vi "CA Spectra.vi"(2 "Header In":T1={"header info"={"Header"="", "Head length"=0}, "A/D info"={"# rf points per line"=0, "# lines per scan"=0, "sample rate MHz"=0, "# A/D bits"=0, "# bytes per A/D"=0, "TGC Flag"=0, "A/D Type"=""}, "Tranducer Info"={"bandwidth"=0.0, "center freq"=0.0, "start freq"=0.0, "ID"=0}, "Scan Info"={"delay"=0.0, "pivot distance"=0.0, "sector scan angle"=0.0, "operator"="", "Scan Mode"="", "location"=""}, "Time/Date Info"={"date"="", "time"=""}, "RF Info"={"RF file name"="", "RF file att"="", "RF cal file name"="", "RF cal file att"=""}, "Patient Info"={"ID"="", "extended ID"="", "age"=0, "sex"="", "previously\nscanned"="", "PSA"=0.0, "LOS"=1, "Ethnicty 2"=3, "Race"=3}, "Tissue Type"={"organ"=0, "disease type"=0, "disease location"=0, "IQ_pts"=0, "RcvBuffer"=0, "RcvFrame"=0, "IQBuff"=0, "IQFrame"=0, "IQPage"=0}, "Votage scaling"={"Digitizer (dB)"=0.0, "Gain (dB)"=0.0, "Atten (dB)"=0.0}, "Comment"="", "Misc Info"={"avg num"=0, "c speed"=0, "Div By or SF zones"=0, "XMIT CHS"=0, "RCV CHS"=0, "Xmit angle"=0.0}, "Therapy Parameters"={"Theraputic Freq (MHz)"=0.1, "Time on (s)"=1.0, "Therapy amplitude (mV)"=50.0, "Lines Before"=20, "Lines After"=80}, "Scan Settings"={"Energy (uJ or V)"=0, "Damp (Ohm) or Fc"=0, "HP Filt (KHz)"=0, "LP Filt (MHz)"=0, "Gain (db)"=0, "prf (kHz)"=0.0, "Distance between\nscan lines (um)"=0, "Distance between\nscan planes (um)"=0, "Scan line gap (um)"=0.0, "Scan plane gap (um)"=0.0}, "Compression Parameters"={"F1 (MHz)"=0.0, "F2 (MHz)"=0.0, "% taper"=0.0, "duration"=0.0}, "Patient Info Xtra"={"First Name"="", "Last Name"="", "Notes"=""}, "ROI Box"=[]} {"Compression Parameters"."% taper" min=50 max=1000 format="%.2f"; "Compression Parameters"."F2 (MHz)" format="%.3f"; "Compression Parameters"."F1 (MHz)" format="%.3f"; "Scan Settings"."prf (kHz)" format="%.2f"; "Therapy Parameters"."Therapy amplitude (mV)" min=50 max=1000 format="%.2f"; "Therapy Parameters"."Time on (s)" format="%.3f"; "Therapy Parameters"."Theraputic Freq (MHz)" format="%.3f"; "Patient Info"."Race" items=["Am Ind or Alaska", "Asian", "Hawaiian, Pac Isl", "Black or Afr Amer", "White", "more than one race", "unknown"]; "Patient Info"."Ethnicty 2" items=["Hispanic", "Non-Hispanic", "unknown"]; "Patient Info"."LOS" items=["1", "2", "3", "4", "5"]; "Patient Info"."PSA" format="%.1f"; "Scan Info"."delay" format="%.2f"; "Scan Info"."pivot distance" format="%.2f"; "Scan Info"."sector scan angle" format="%.2f"; "Tranducer Info"."bandwidth" format="%.2f"; "Tranducer Info"."center freq" format="%.2f"; "Tranducer Info"."start freq" format="%.2f"}, 3 "time array":u32[](array[numeric]), 5 "Data in":dbl[][](array[numeric]), 6 "2nd freq":dbl=20.0, 8 "Excitation Type":u16(ring)=1 items=["tone burst", "chirp"], 12 "sub thresh":dbl=32.0) -> (7 "Windowed RF traces":dbl[][](array[numeric]), 11 "sub time":cluster{i32[], "Best Linear Fit":dbl[]}[](graph), 13 "ratio histo":T3(graph), 14 "Spectra":cluster{i32, "df":dbl, dbl[][]}(graph), 15 "output params":T2 {"r^2 sub" format="%#.6g"; "slope sub" format="%#.6g"; "r^2 cum" format="%#.6g"; "slope cum" format="%#.6g"}, 17 "Sub indexes":dbl[](array[numeric]), 18 "total time":cluster{i32[], "Best Linear Fit":dbl[]}[](graph), 19 "Scatter":cluster{dbl[], "Best Linear Fit":dbl[]}[](graph))   [LabVIEW 2022 SP3]
uses:
  ViewData/-ReadEye/Header.ctl
  <vilib>/Analysis/2dsp.llb/1D Convolution (DBL).vi
  <vilib>/Analysis/4window.llb/Hamming Window (DBL).vi
  <vilib>/Analysis/4window.llb/AllCosWindow (DBL).vi
  <vilib>/Analysis/2dsp.llb/1D Cross Correlation (DBL).vi
  <vilib>/Analysis/NI_AALBase.lvlib
  <vilib>/Analysis/NI_AALPro.lvlib
  <vilib>/gmath/NI_Gmath.lvlib
panel:
  in  "MSE Thresh":dbl=0.1
  out "ASub dB":dbl[](array[numeric])
  out "Linear spec":T4(graph)
  in  "FFT size":u16(ring)=9 items=["next 2^n", "8", "16", "32", "64", "128", "256", "512", "1024", "2048"]
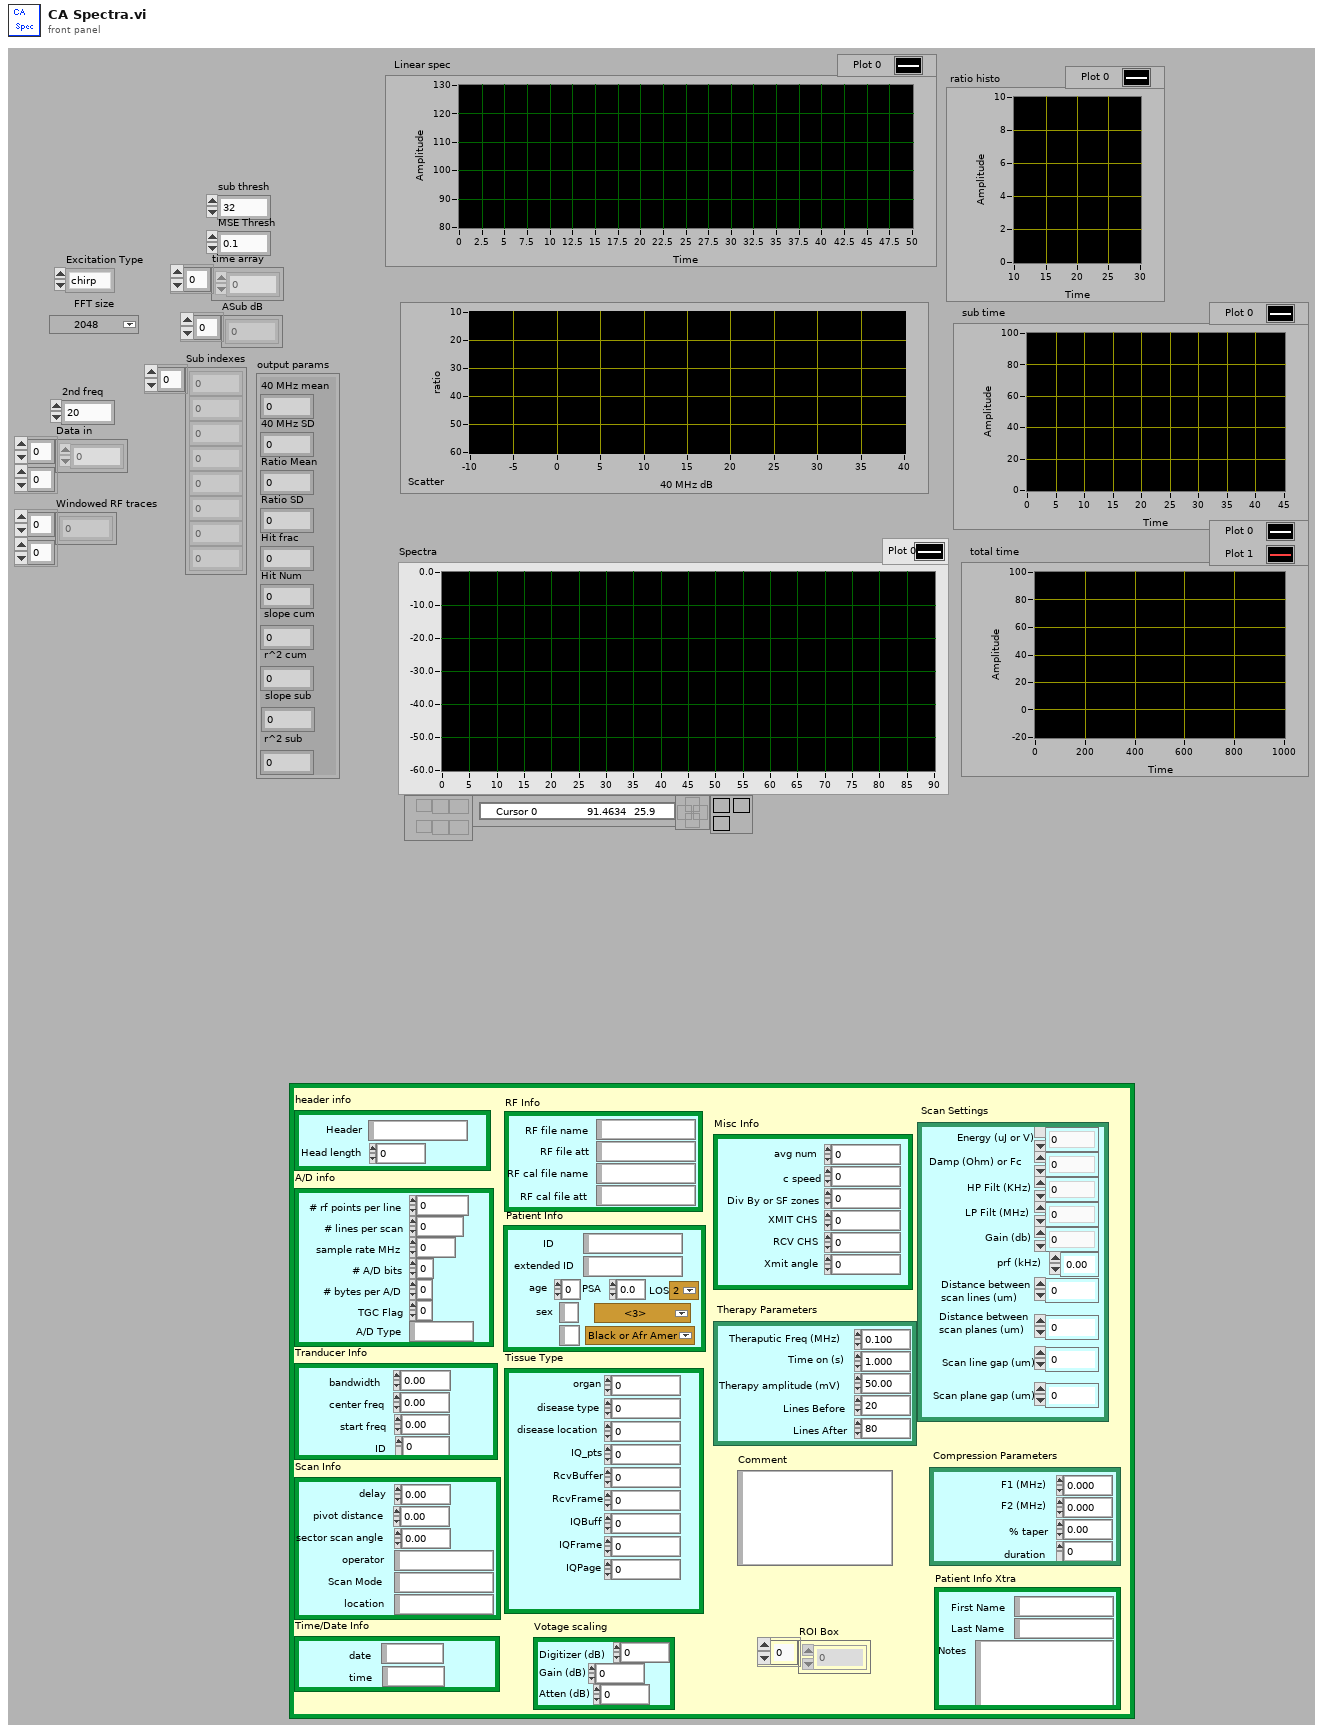
[diagram p1: front panel]
types:
  T1 = typedef "Header.ctl" = cluster{"header info":cluster{"Header":string, "Head length":i16}, "A/D info":cluster{"# rf points per line":u16, "# lines per scan":u16, "sample rate MHz":u16, "# A/D bits":i16, "# bytes per A/D":u16, "TGC Flag":u16, "A/D Type":string}, "Tranducer Info":cluster{"bandwidth":sgl, "center freq":sgl, "start freq":sgl, "ID":i32}, "Scan Info":cluster{"delay":sgl, "pivot distance":sgl, "sector scan angle":sgl, "operator":string, "Scan Mode":string, "location":string}, "Time/Date Info":cluster{"date":string, "time":string}, "RF Info":cluster{"RF file name":string, "RF file att":string, "RF cal file name":string, "RF cal file att":string}, "Patient Info":cluster{"ID":string, "extended ID":string, "age":u16, "sex":string, "previously\nscanned":string, "PSA":sgl, "LOS":u8, "Ethnicty 2":u8, "Race":u8}, "Tissue Type":cluster{"organ":i16, "disease type":i16, "disease location":i16, "IQ_pts":u16, "RcvBuffer":u8, "RcvFrame":u16, "IQBuff":u8, "IQFrame":u16, "IQPage":u8}, "Votage scaling":cluster{"Digitizer (dB)":sgl, "Gain (dB)":sgl, "Atten (dB)":sgl}, "Comment":string, "Misc Info":cluster{"avg num":u16, "c speed":i16, "Div By or SF zones":i16, "XMIT CHS":u8, "RCV CHS":u8, "Xmit angle":sgl}, "Therapy Parameters":cluster{"Theraputic Freq (MHz)":sgl, "Time on (s)":sgl, "Therapy amplitude (mV)":sgl, "Lines Before":u16, "Lines After":u16}, "Scan Settings":cluster{"Energy (uJ or V)":u8, "Damp (Ohm) or Fc":u8, "HP Filt (KHz)":u8, "LP Filt (MHz)":u8, "Gain (db)":u8, "prf (kHz)":sgl, "Distance between\nscan lines (um)":u16, "Distance between\nscan planes (um)":u16, "Scan line gap (um)":sgl, "Scan plane gap (um)":sgl}, "Compression Parameters":cluster{"F1 (MHz)":sgl, "F2 (MHz)":sgl, "% taper":sgl, "duration":sgl}, "Patient Info Xtra":cluster{"First Name":string, "Last Name":string, "Notes":string}, "ROI Box":u16[]}
  T2 = cluster{"40 MHz mean":dbl, "40 MHz SD":dbl, "Ratio Mean":dbl, "Ratio SD":dbl, "Hit frac":dbl, "Hit Num":i32, "slope cum":dbl, "r^2 cum":dbl, "slope sub":dbl, "r^2 sub":dbl}
  T3 = cluster{"X Values":dbl[], "Histogram: h(x)":i32[]}
  T4 = cluster{i32, "df":dbl, "Power Spectrum (V^2 rms)":dbl[]}
  T5 = cluster{"mean":dbl, "standard deviation":dbl, "mean":dbl, "standard deviation":dbl, dbl, i32, "slope":dbl, "r^2":dbl, "slope":dbl, "r^2":dbl}
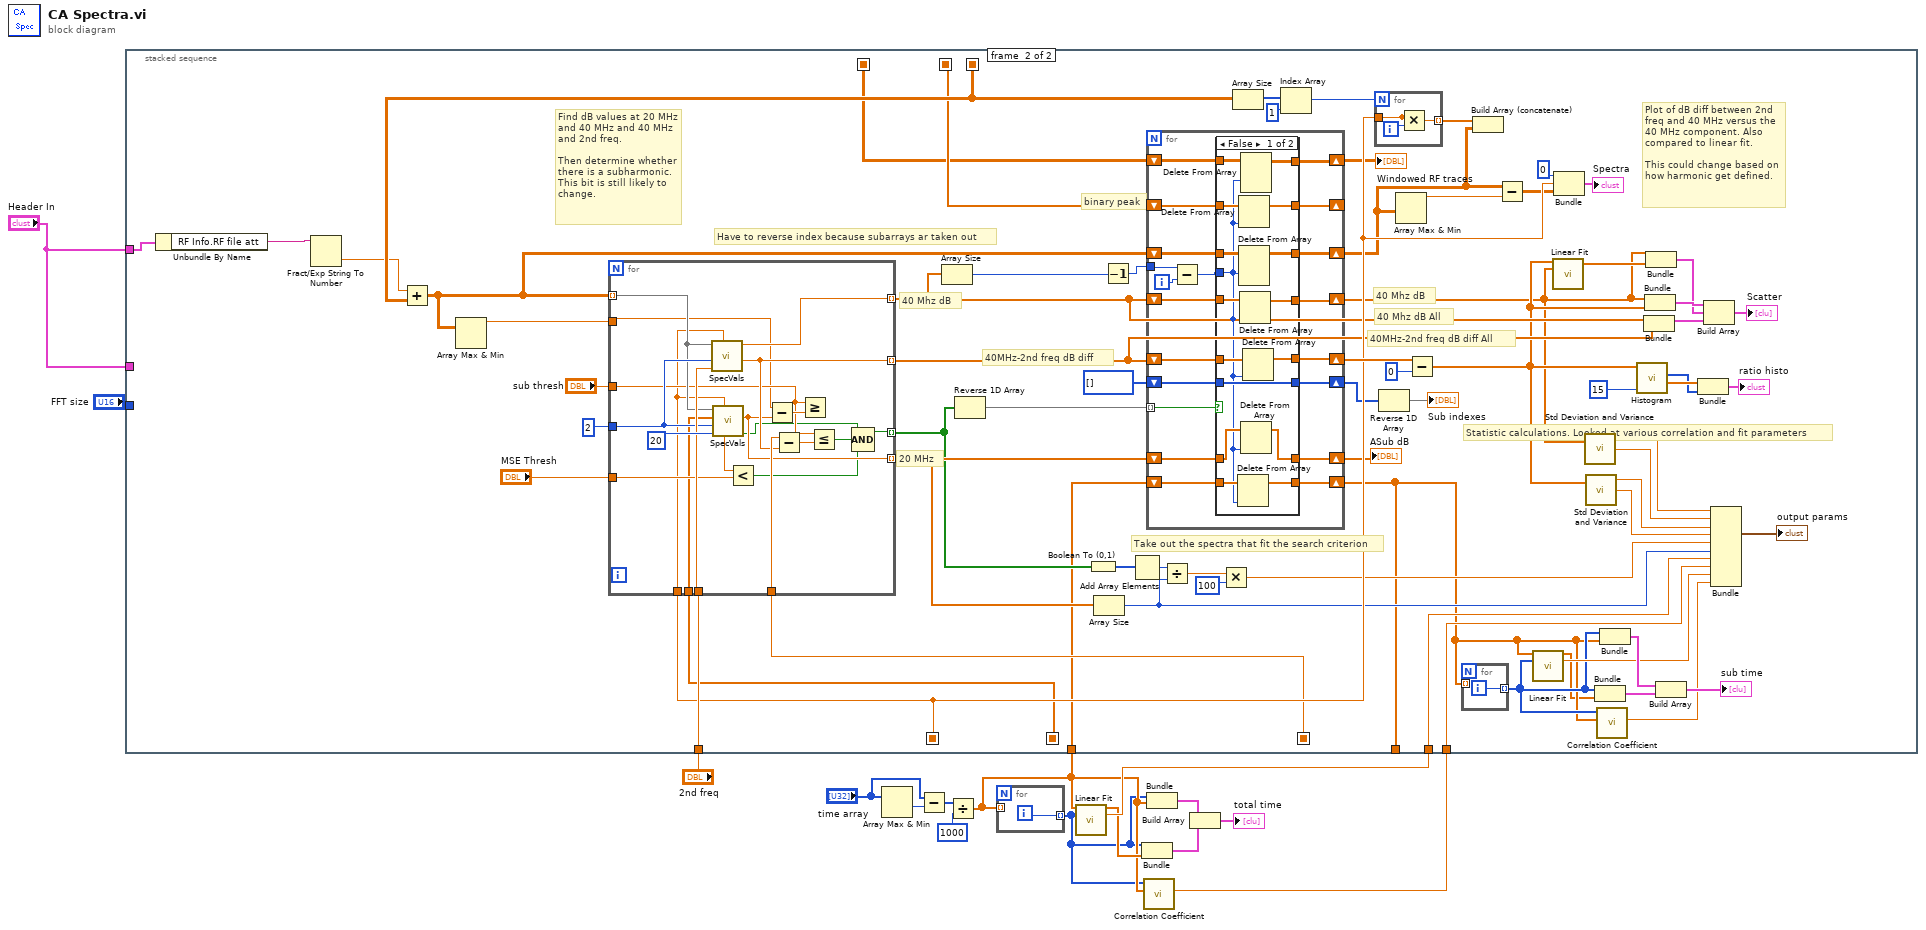
[diagram p0: block diagram]
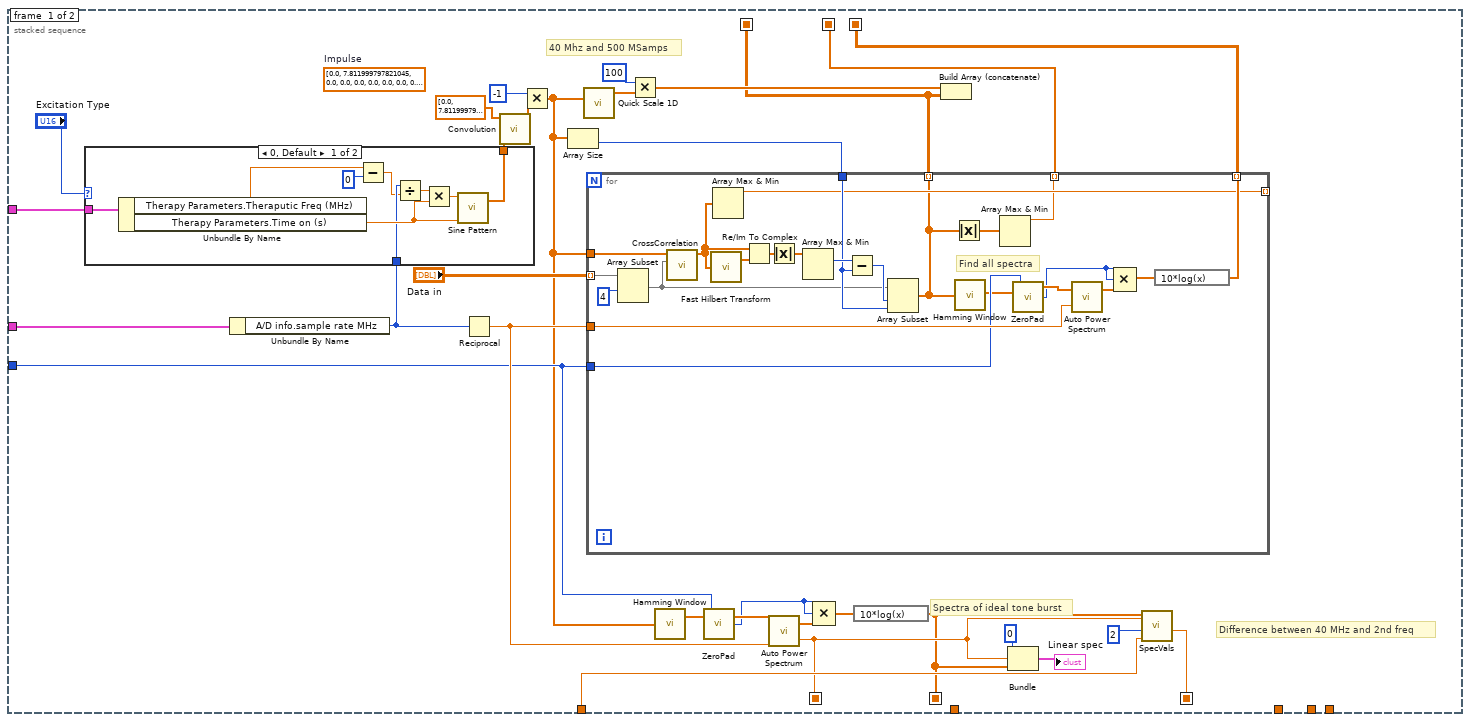
[diagram p2: hidden frame]
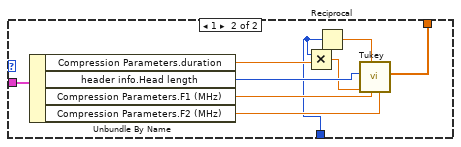
[diagram p3: hidden frame]
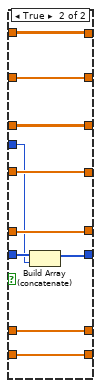
[diagram p4: hidden frame]
diagram:
  n1 = Array Max & Min(array="time array") -> (min value=w13:u32)  [unwired: 3 out]
  n2 = Subtract(x="time array", y=w13) -> (x-y=w11:u32[])
  n3 = Divide(x=w11, y=1000) -> (x/y=w4:dbl[])
  n4 = for {
    tunnel: w4 -> [_] mode=indexing
    tunnel: [w16] -> w3 mode=indexing
    i -> [w16]
  }
  n5 = call <vilib>:"Linear Fit.vi"("Y"=w4, "X"=w3) -> ("Best Linear Fit"=w5:dbl[], "slope"=w6:dbl)  [unwired: 4 in, 8 out]
  n6 = Bundle(w3, "Best Linear Fit"=w5) -> (w9:cluster{i32[], "Best Linear Fit":dbl[]})  [unwired: 1 out]
  n7 = call <vilib>:"Correlation Coefficient.vi"("Y"=w4, "X"=w3) -> ("r^2"=w2:dbl)  [unwired: 9 out]
  n8 = stacked-sequence {
    seq-local: [w32 _] -> [_ w138]
    seq-local: [w26 _] -> [_ w134]
    seq-local: [w29 _] -> [_ w127]
    seq-local: [w25 _] -> [_ w120]
    seq-local: [w24 _] -> [_ w122]
    seq-local: [w20 _] -> [_ w108]
    tunnel: "2nd freq" -> [w31 w155]
    tunnel: "FFT size" -> [w22 _]
    tunnel: w4 -> [_ w105]
    tunnel: [_ w96] -> _
    tunnel: w6 -> [_ w104]
    tunnel: w2 -> [_ w103]
    tunnel: "Header In" -> [w18 _]
    tunnel: "Header In" -> [w17 w91]
    frame #0 {
      (unwired) sgl[] [0.0, 7.812, 0.0, 0.0, 0.0, 0.0, 0.0, 0.0, 0.0, 0.0, 0.0, -7.812, -31.25, -39.062, -62.5, -93.75, -101.562, -78.125, -15.625, 93.75, 234.375, 367.187, 445.312, 437.5, 351.562, 156.25, -70.312, -289.062, -460.937, -546.875, -562.5, -500.0, -335.937, -78.125, 257.812, 546.875, 734.375, 757.812, 593.75, 320.312, 0.0, -273.437, -437.5, -468.75, -421.875, -296.875, -156.25, 15.625, 164.062, 265.625, 296.875, 257.812, 179.687, 85.937, -7.812, -78.125, -125.0, -140.625, -125.0, -93.75, -54.687, -7.812, 31.25, 62.5, 70.312, 70.312, 54.687, 39.062, 15.625, 0.0, -15.625, -23.437, -23.437, -23.437, -23.437, -15.625, -7.812, 7.812, 7.812, 15.625, 23.437, 23.437, 15.625, 15.625, 15.625, 0.0, 0.0, 0.0, -23.437, -15.625, -15.625, 0.0, 0.0, 7.812, 15.625, 23.437, 15.625, 7.812, 7.812, 0.0, -7.812, -7.812, -15.625, -15.625, -7.812, 0.0, 7.812, 7.812, 15.625, 15.625, 7.812, 7.812, 0.0, -7.812, 0.0, -7.812, 0.0, -7.812, 0.0, 0.0, 0.0, 7.812, 7.812, 7.812, 7.812, 0.0, 0.0, 0.0, 0.0, 0.0]  # Impulse
      # "Difference between 40 MHz and 2nd freq"
      # "Spectra of ideal tone burst"
      # "40 Mhz and 500 MSamps"
      n9 = Unbundle By Name(w18) -> ("A/D info.sample rate MHz"=w37:u16)
      n10 = case shown="0, Default" "Excitation Type" {
        tunnel: [w56 w58] -> w43
        tunnel: w37 -> [w52 w59]
        tunnel: w17 -> [w48 w57]
        frame 0, Default {
          n11 = Unbundle By Name(w48) -> ("Therapy Parameters.Theraputic Freq (MHz)"=w51:sgl, "Therapy Parameters.Time on (s)"=w55:sgl)
          n12 = Subtract(x=w51, y=0) -> (x-y=w50:sgl)
          n13 = Divide(x=w52, y=w50) -> (x/y=w54:sgl)
          n14 = Multiply(x=w54, y=w55) -> (x*y=w53:sgl)
          n15 = call <vilib>:"Sine Pattern.vi"("cycles"=w55, "samples"=w53) -> ("Sinusoidal Pattern"=w56:dbl[])  [unwired: 2 in, 1 out]
        }
        frame 1 {
          n16 = Unbundle By Name(w57) -> ("Compression Parameters.duration"=w60:sgl, "header info.Head length"=w65:i16, "Compression Parameters.F1 (MHz)"=w61:sgl, "Compression Parameters.F2 (MHz)"=w62:sgl)
          n17 = Multiply(x=w59, y=w60) -> (x*y=w64:sgl)
          n18 = Reciprocal(x=w59) -> (1/x=w63:dbl)
          n19 = call "Tukey.vi"("f2 (MHz)"=w62, "f1 (MHz)"=w61, "Samp Rate (mics)"=w63, "Pts"=w64, "Tukey"=w65) -> ("Tukey Chirp"=w58:dbl[])  [unwired: 2 in, 4 out]
        }
      }
      n20 = Reciprocal(x=w37) -> (1/x=w36:dbl)
      n21 = call-poly <vilib>:"Convolution.vi"("Y"=w43, "X"=sgl[] [0.0, 7.812, 7.812, 0.0, 0.0, -15.625, -31.25, -46.875, -31.25, 31.25, 132.812, 257.812, 328.125, 304.687, 179.687, -31.25, -257.812, -421.875, -484.375, -468.75, -406.25, -289.062, -93.75, 210.937, 562.5, 812.5, 851.562, 664.062, 250.0, -210.937, -578.125, -742.187, -703.125, -484.375, -218.75, 31.25, 281.25, 468.75, 515.625, 421.875, 210.937, -39.062, -218.75, -304.687, -296.875, -218.75, -101.562, 0.0, 109.375, 187.5, 218.75, 195.312, 132.812, 54.687, -7.812, -54.687, -70.312, -62.5, -31.25, 0.0, 39.062, 62.5, 85.937, 93.75, 78.125, 46.875, 23.437, -7.812, -15.625, -15.625, -23.437, -15.625, 7.812, 7.812, 15.625, 31.25, 15.625, 15.625, 7.812, 0.0, -7.812, -7.812, -7.812, 0.0, -7.812] ("decimated array")) -> ("X * Y"=w28:dbl[])  [unwired: 1 in, 8 out]
      n22 = Multiply(x=-1, y=w28) -> (x*y=w21:dbl[])
      n23 = Array Size(array=w21) -> (size(s)=w47:i32)
      n24 = call <vilib>:"Quick Scale 1D.vi"("X"=w21) -> ("Y[i]=X[i]/Max|X|"=w44:dbl[])  [unwired: 2 out]
      n25 = for {
        tunnel: "Data in" -> [w86] mode=indexing
        tunnel: w21 -> [w88]
        tunnel: [w79] -> w32 mode=indexing
        tunnel: [w66] -> w25 mode=indexing
        tunnel: w47 -> [w82]
        tunnel: w22 -> [w77]
        tunnel: w36 -> [w80]
        tunnel: [w78] -> _ mode=indexing
        tunnel: [w72] -> w24 mode=indexing
        # "Find all spectra"
        n26 = Array Subset(array=w86, index=4) -> (w67:dbl[])  [unwired: 1 in]
        n27 = call-poly <vilib>:"CrossCorrelation.vi"("Y"=w67, "X"=w88) -> ("Rxy"=w69:dbl[])  [unwired: 2 in, 7 out]
        n28 = call <vilib>:"Fast Hilbert Transform.vi"("X"=w69) -> ("Hilbert{X}"=w84:dbl[])  [unwired: 1 out]
        n29 = Array Max & Min(array=w69) -> (max value=w78:dbl)  [unwired: 3 out]
        n30 = Re/Im To Complex(1:w84, 2:w69) -> (0:w83:cdb[])
        n31 = Absolute Value(x=w83) -> (abs(x)=w70:dbl[])
        n32 = Array Max & Min(array=w70) -> (max index (indices)=w87:i32)  [unwired: 3 out]
        n33 = Subtract(x=w87, y=w82) -> (x-y=w68:i32)
        n34 = Array Subset(array=w67, index=w68, length=w82) -> (w66:dbl[])
        n35 = Absolute Value(x=w66) -> (abs(x)=w73:dbl[])
        n36 = call-poly <vilib>:"Hamming Window.vi"("X"=w66) -> ("Windowed X"=w71:dbl[])  [unwired: 1 out]
        n37 = Array Max & Min(array=w73) -> (max value=w72:dbl)  [unwired: 3 out]
        n38 = call "ZeroPad.vi"("Input Array"=w71, "FFT size"=w77) -> ("Length of padded array"=w75:i32, "Ouput Array"=w76:dbl[])  [unwired: 3 out]
        n39 = call <vilib>:"Auto Power Spectrum.vi"("dt"=w80, "Signal (V)"=w76) -> ("Power Spectrum (V^2 rms)"=w81:dbl[])  [unwired: 1 out]
        n40 = Compound Arithmetic op=MULTIPLY(w75, w75, w81) -> (w74:dbl[])
        n41 = expression code="10*log(x)"(w74) -> (w79:dbl[])
      }
      n42 = Multiply(x=100, y=w44) -> (x*y=w41:dbl[])
      n43 = call-poly <vilib>:"Hamming Window.vi"("X"=w21) -> ("Windowed X"=w38:dbl[])  [unwired: 1 out]
      n44 = call "ZeroPad.vi"("Input Array"=w38, "FFT size"=w22) -> ("Length of padded array"=w34:i32, "Ouput Array"=w42:dbl[])  [unwired: 3 out]
      n45 = call <vilib>:"Auto Power Spectrum.vi"("dt"=w36, "Signal (V)"=w42) -> ("df"=w26:dbl, "Power Spectrum (V^2 rms)"=w35:dbl[])
      n46 = Compound Arithmetic op=MULTIPLY(w34, w34, w35) -> (w33:dbl[])
      n47 = expression code="10*log(x)"(w33) -> (w20:dbl[])
      n48 = Build Array (concatenate)(w41, w25) -> ()  [unwired: 1 out]
      n49 = Bundle(0, "df"=w26, w20) -> (→"Linear spec":cluster{i32, "df":dbl, dbl[]})  [unwired: 1 out]
      n50 = call "SpecVals.vi"("df"=w26, "2nd freq"=w31, "window"=2, "Power Spectrum"=w20) -> ("diff"=w29:dbl)  [unwired: 1 in, 4 out]
    }
    frame #1 {
      # "40MHz-2nd freq dB diff All"
      # "40 Mhz dB All"
      # "40 Mhz dB"
      # "binary peak"
      # "Have to reverse index because subarrays ar taken out"
      # "Plot of dB diff between 2nd freq and 40 MHz versus the 40 MHz component. Also compared to linear fit.\n\nThis could change based on how harmonic get defined."
      # "40MHz-2nd freq dB diff"
      # "40 Mhz dB"
      # "Statistic calculations. Looked at various correlation and fit parameters"
      # "Take out the spectra that fit the search criterion"
      # "Find dB values at 20 MHz and 40 MHz and 40 MHz and 2nd freq. \n\nThen determine whether there is a subharmonic. This bit is still likely to change."
      # "20 MHz"
      n51 = Unbundle By Name(w91) -> ("RF Info.RF file att"=w90:string)
      n52 = Fract/Exp String To Number(string=w90) -> (number=w89:dbl)  [unwired: 4 out]
      n53 = Add(x=w89, y=w138) -> (x+y=w133:dbl[][])
      n54 = Array Max & Min(array=w133) -> (max value=w119:dbl)  [unwired: 3 out]
      n55 = for {
        tunnel: [w226] -> w121 mode=indexing
        tunnel: [w221] -> w124 mode=indexing
        tunnel: w155 -> [w228]
        tunnel: w133 -> [w225] mode=indexing
        tunnel: w134 -> [w210]
        tunnel: "sub thresh" -> [w220]
        tunnel: 2 -> [w227]
        tunnel: [w216] -> w144 mode=indexing
        tunnel: w119 -> [w217]
        tunnel: w127 -> [w223]
        tunnel: [w215] -> w118 mode=indexing
        tunnel: "MSE Thresh" -> [w219]
        tunnel: w108 -> [w218]
        n56 = call "SpecVals.vi"("df"=w210, "2nd freq"=w228, "window"=w227, "Power Spectrum"=w225) -> ("diff"=w221:dbl, "40 Mhz db"=w226:dbl)  [unwired: 1 in, 3 out]
        n57 = call "SpecVals.vi"("df"=w210, "2nd freq"=20, "window"=w227, "Tone Burst"=w218, "Power Spectrum"=w225) -> ("x < 0?"=w212:bool, "2nd f db"=w216:dbl, "MSE"=w211:dbl)  [unwired: 2 out]
        n58 = Less?(x=w211, y=w219) -> (x < y?=w213:bool)
        n59 = Subtract(x=w217, y=w216) -> (x-y=w224:dbl)
        n60 = Subtract(x=w223, y=w221) -> (x-y=w222:dbl)
        n61 = Greater Or Equal?(x=w220, y=w224) -> ()  [unwired: 1 out]
        n62 = Less Or Equal?(x=w220, y=w222) -> (x <= y?=w214:bool)
        n63 = Compound Arithmetic op=AND(w212, w214, w213) -> (w215:bool)
      }
      n64 = Array Size(array=w121) -> (size(s)=w139:i32)
      n65 = Reverse 1D Array(array=w118) -> (reversed array=w130:bool[])
      n66 = Boolean To (0,1)(Boolean=w118) -> (0, 1=w143:i16[])
      n67 = Array Size(array=w144) -> (size(s)=w111:i32)
      n68 = Decrement(x=w139) -> (x-1=w154:i32)
      n69 = Add Array Elements(numeric array=w143) -> (sum=w142:i16)
      n70 = for {
        tunnel: w130 -> [w180] mode=indexing
        tunnel: w154 -> [w183]
        shift-right: [w176] -> w107
        shift-left: w121 -> [w177]
        shift-right: [w175] -> w152
        shift-left: w124 -> [w178]
        shift-right: [w181] -> w93
        shift-left: w133 -> [w182]
        shift-right: [w174] -> w128
        shift-left: w144 -> [w179]
        shift-right: [w172] -> w126
        shift-left: w120 -> [w173]
        shift-right: [w171] -> w131
        shift-left: i32[] [] -> [w170]
        shift-right: [w166] -> _
        shift-left: w122 -> [w167]
        shift-right: [w164] -> w96
        shift-left: w105 -> [w165]
        i -> [w169]
        n71 = Subtract(x=w183, y=w169) -> (x-y=w168:i32)
        n72 = case shown="False" w180 {
          tunnel: w182 -> [w199 w209]
          tunnel: [w198 w209] -> w181
          tunnel: w168 -> [w184 w202]
          tunnel: w179 -> [w187 w206]
          tunnel: w178 -> [w197 w207]
          tunnel: w177 -> [w196 w208]
          tunnel: [w195 w208] -> w176
          tunnel: [w194 w207] -> w175
          tunnel: [w193 w206] -> w174
          tunnel: w173 -> [w192 w205]
          tunnel: [w191 w205] -> w172
          tunnel: [w190 w203] -> w171
          tunnel: w170 -> [w190 w204]
          tunnel: [w188 w201] -> w166
          tunnel: w167 -> [w189 w201]
          tunnel: w165 -> [w186 w200]
          tunnel: [w185 w200] -> w164
          frame False {
            n73 = Delete From Array(array=w186, index=w184) -> (array with subset deleted=w185:dbl[])  [unwired: 1 in, 1 out]
            n74 = Delete From Array(array=w189, index=w184) -> (array with subset deleted=w188:dbl[])  [unwired: 1 in, 1 out]
            n75 = Delete From Array(array=w199, index (row)=w184) -> (array with subset deleted=w198:dbl[][])  [unwired: 2 in, 1 out]
            n76 = Delete From Array(array=w196, index=w184) -> (array with subset deleted=w195:dbl[])  [unwired: 1 in, 1 out]
            n77 = Delete From Array(array=w192, index (row)=w184) -> (array with subset deleted=w191:dbl[][])  [unwired: 2 in, 1 out]
            n78 = Delete From Array(array=w187, index=w184) -> (array with subset deleted=w193:dbl[])  [unwired: 1 in, 1 out]
            n79 = Delete From Array(array=w197, index=w184) -> (array with subset deleted=w194:dbl[])  [unwired: 1 in, 1 out]
          }
          frame True {
            n80 = Build Array (concatenate)(w204, w202) -> (w203:i32[])
          }
        }
      }
      "Windowed RF traces" <- w126
      "ASub dB" <- w128
      n81 = Divide(x=w142, y=w111) -> (x/y=w140:dbl)
      n82 = Multiply(x=w140, y=100) -> (x*y=w112:dbl)
      n83 = Array Size(array=w138) -> (size(s)=w137:i32[])
      n84 = Index Array(array=w137, index=1) -> (element=w135:i32)
      n85 = for {
        N: w135 -> [_]
        tunnel: [w163] -> w109 mode=indexing
        tunnel: [w161] -> _ mode=indexing
        tunnel: w134 -> [w161]
        i -> [w162]
        n86 = Multiply(x=w161, y=w162) -> (x*y=w163:dbl)
      }
      n87 = Reverse 1D Array(array=w131) -> (reversed array=→"Sub indexes":i32[])
      n88 = Array Max & Min(array=w93) -> (max value=w94:dbl)  [unwired: 3 out]
      n89 = Subtract(x=w152, y=0) -> (x-y=w115:dbl[])
      n90 = for {
        tunnel: [w160] -> w98 mode=indexing
        tunnel: w96 -> [_] mode=indexing
        i -> [w160]
      }
      n91 = Build Array (concatenate)(w109, w93) -> ()  [unwired: 1 out]
      n92 = Subtract(x=w93, y=w94) -> (x-y=w92:dbl[][])
      n93 = call <vilib>:"Linear Fit.vi"("Y"=w96, "X"=w98) -> ("Best Linear Fit"=w95:dbl[], "slope"=w99:dbl)  [unwired: 4 in, 8 out]
      n94 = call <vilib>:"Linear Fit.vi"("Y"=w115, "X"=w107) -> ("Best Linear Fit"=w158:dbl[])  [unwired: 4 in, 9 out]
      n95 = Bundle(0, "df"=w134, w92) -> (→"Spectra":cluster{i32, "df":dbl, dbl[][]})  [unwired: 1 out]
      n96 = call <vilib>:"Std Deviation and Variance.vi"("X"=w107) -> ("mean"=w117:dbl, "standard deviation"=w116:dbl)  [unwired: 1 in, 1 out]
      n97 = call <vilib>:"Std Deviation and Variance.vi"("X"=w115) -> ("mean"=w114:dbl, "standard deviation"=w113:dbl)  [unwired: 1 in, 1 out]
      n98 = Bundle(w98, "Best Linear Fit"=w95) -> (w101:cluster{i32[], "Best Linear Fit":dbl[]})  [unwired: 1 out]
      n99 = call <vilib>:"Correlation Coefficient.vi"("Y"=w96, "X"=w98) -> ("r^2"=w97:dbl)  [unwired: 9 out]
      n100 = Bundle(w98, w96) -> (w100:cluster{i32[], dbl[]})  [unwired: 1 out]
      n101 = call <vilib>:"Histogram.vi"("intervals"=15, "X"=w115) -> ("X Values"=w148:dbl[], "Histogram: h(x)"=w147:i32[])  [unwired: 8 out]
      n102 = Bundle(w121, w124) -> (w123:cluster{dbl[], dbl[]})  [unwired: 1 out]
      n103 = Bundle(w107, w115) -> (w156:cluster{dbl[], dbl[]})  [unwired: 1 out]
      n104 = Bundle(w107, "Best Linear Fit"=w158) -> (w153:cluster{dbl[], "Best Linear Fit":dbl[]})  [unwired: 1 out]
      n105 = Build Array(w100, w101) -> (→"sub time":cluster{i32[], "Best Linear Fit":dbl[]}[])
      n106 = Bundle("X Values"=w148, "Histogram: h(x)"=w147) -> (→"ratio histo":T3)  [unwired: 1 out]
      n107 = Build Array(w156, w153, w123) -> (→"Scatter":cluster{dbl[], "Best Linear Fit":dbl[]}[])
      n108 = Bundle("mean"=w117, "standard deviation"=w116, "mean"=w114, "standard deviation"=w113, w112, w111, "slope"=w104, "r^2"=w103, "slope"=w99, "r^2"=w97) -> (→"output params":T5)  [unwired: 1 out]
    }
  }
  n109 = Bundle(w3, w4) -> (w10:cluster{i32[], dbl[]})  [unwired: 1 out]
  n110 = Build Array(w10, w9) -> (→"total time":cluster{i32[], "Best Linear Fit":dbl[]}[])
